vi "Read Encoders From Registry (Internal).vi"(8 "error in (no error)":errorcluster, 10 "CMD LUT":variant) -> (0 "error out":errorcluster, 2 "Encoders":T1[](array[typedef]) {"Encoder Filter" max=255; "Backlash Period (s)" min=0.0005 max=10.0 step=0.0005; "Multiplier" min=1 max=100000; "Counts/mm" min=1 max=100000})   [LabVIEW 2026, in "MicroPulse_Driver.lvlib"]
uses:
  MicroPulse_Driver.lvlib
  Public/Data/Datatypes/MP - encoder settings.ctl
  Public/Data/Datatypes/MP - encoder type.ctl
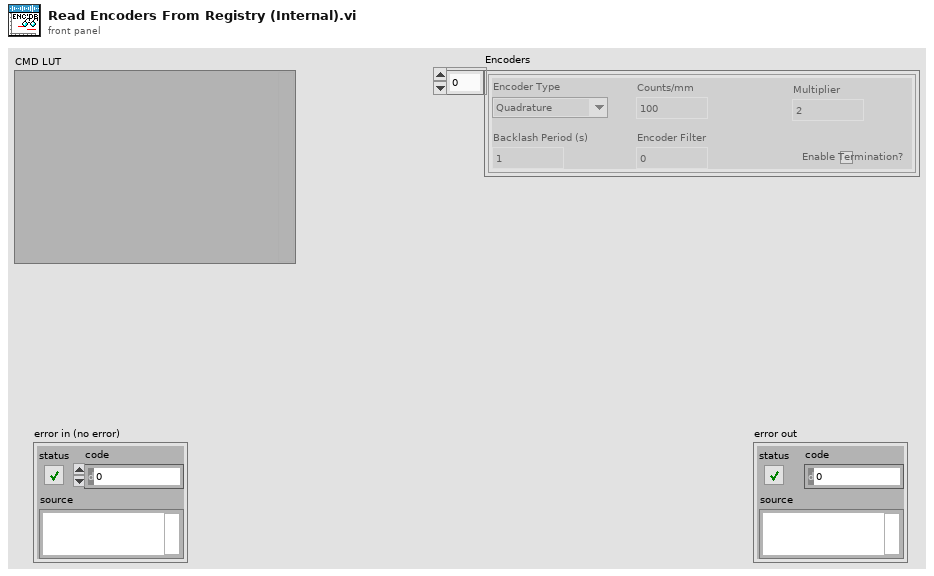
[diagram p1: front panel]
types:
  T1 = typedef "MicroPulse_Driver.lvlib/MP - encoder settings.ctl" = cluster{"Encoder Type":T2, "Counts/mm":u32, "Enable Termination?":bool, "Multiplier":u32, "Backlash Period (s)":dbl, "Encoder Filter":u32}
  T2 = typedef "MicroPulse_Driver.lvlib/MP - encoder type.ctl" = enum16{"Quadrature", "Step/Direction"}
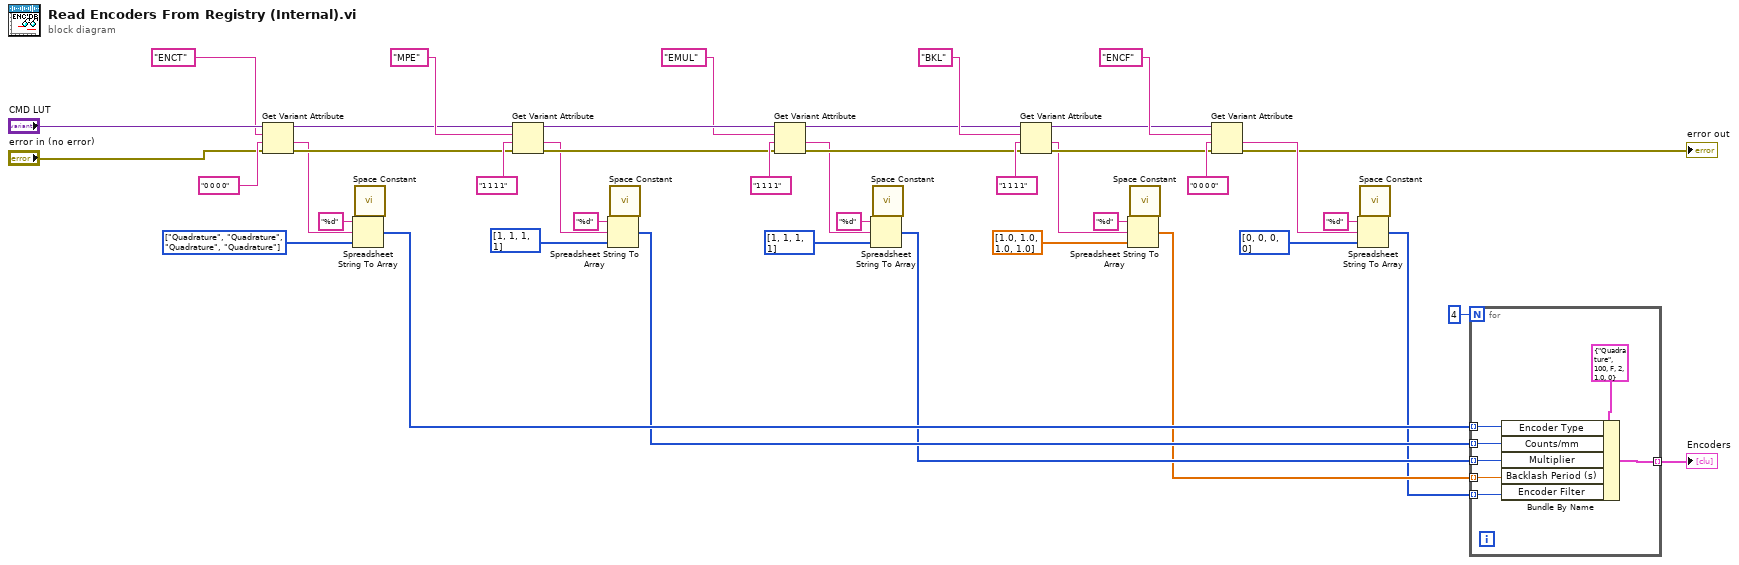
[diagram p0: block diagram]
diagram:
  w27 = T2[] [enum."Quadrature", enum."Quadrature", enum."Quadrature", enum."Quadrature"] items=["Quadrature", "Step/Direction"] ("Array")
  n1 = Get Variant Attribute(Variant="CMD LUT", name="ENCT", default value (empty Variant)="0 0 0 0", error in="error in (no error)") -> (duplicate Variant=w34:variant, value=w26:string, error out=w36:errorcluster)  [unwired: 1 out]
  n2 = call <vilib>:"Space Constant.vi"() -> ("String"=w28:string)
  n3 = Spreadsheet String To Array(delimiter (Tab)=w28, format string="%d", spreadsheet string=w26, array type (2D Dbl)=w27) -> (array=w9:T2[])
  n4 = Get Variant Attribute(Variant=w34, name="MPE", default value (empty Variant)="1 1 1 1", error in=w36) -> (duplicate Variant=w47:variant, value=w16:string, error out=w39:errorcluster)  [unwired: 1 out]
  n5 = call <vilib>:"Space Constant.vi"() -> ("String"=w25:string)
  n6 = Spreadsheet String To Array(delimiter (Tab)=w25, format string="%d", spreadsheet string=w16, array type (2D Dbl)=u32[] [1, 1, 1, 1] ("Counts/mm")) -> (array=w8:u32[])
  n7 = Get Variant Attribute(Variant=w47, name="EMUL", default value (empty Variant)="1 1 1 1", error in=w39) -> (duplicate Variant=w41:variant, value=w14:string, error out=w40:errorcluster)  [unwired: 1 out]
  n8 = call <vilib>:"Space Constant.vi"() -> ("String"=w22:string)
  n9 = Spreadsheet String To Array(delimiter (Tab)=w22, format string="%d", spreadsheet string=w14, array type (2D Dbl)=u32[] [1, 1, 1, 1] ("Multiplier")) -> (array=w7:u32[])
  n10 = Get Variant Attribute(Variant=w41, name="BKL", default value (empty Variant)="1 1 1 1", error in=w40) -> (duplicate Variant=w31:variant, value=w12:string, error out=w30:errorcluster)  [unwired: 1 out]
  n11 = call <vilib>:"Space Constant.vi"() -> ("String"=w21:string)
  n12 = Spreadsheet String To Array(delimiter (Tab)=w21, format string="%d", spreadsheet string=w12, array type (2D Dbl)=dbl[] [1.0, 1.0, 1.0, 1.0] ("Backlash Period (s)")) -> (array=w6:dbl[])
  n13 = Get Variant Attribute(Variant=w31, name="ENCF", default value (empty Variant)="0 0 0 0", error in=w30) -> (value=w10:string, error out=→"error out":errorcluster)  [unwired: 2 out]
  n14 = call <vilib>:"Space Constant.vi"() -> ("String"=w18:string)
  n15 = Spreadsheet String To Array(delimiter (Tab)=w18, format string="%d", spreadsheet string=w10, array type (2D Dbl)=u32[] [0, 0, 0, 0] ("Encoder Filter")) -> (array=w5:u32[])
  n16 = for {
    N: 4 -> [_]
    tunnel: w9 -> [w54] mode=indexing
    tunnel: w8 -> [w53] mode=indexing
    tunnel: w7 -> [w52] mode=indexing
    tunnel: w6 -> [w51] mode=indexing
    tunnel: w5 -> [w50] mode=indexing
    tunnel: [w49] -> w2 mode=indexing
    n17 = Bundle By Name(cluster=T1 {"Encoder Type"=enum."Quadrature", "Counts/mm"=100, "Enable Termination?"=FALSE, "Multiplier"=2, "Backlash Period (s)"=1.0, "Encoder Filter"=0} ("Encoder Settings"), "Encoder Type"=w54, "Counts/mm"=w53, "Multiplier"=w52, "Backlash Period (s)"=w51, "Encoder Filter"=w50) -> (w49:T1)
  }
  "Encoders" <- w2
